vi "Talker.vi"(0 "Divide in":refnum<class "Divide.lvclass">, 5 "Subpanel Ref":refnum<vi>, 11 "Error In":errorcluster) -> (4 "Divide out":refnum<class "Divide.lvclass">, 15 "Error Out":errorcluster)   [LabVIEW 2020, in "Divide.lvclass"]
doc: "Method to call the UI Method. This will pass the object to the UI Method which will do the operation and return the object to the main vi."
uses:
  Divide.lvclass
  D:/Github Projects/LV_Assignment/Tasks/A18/A18/Classes/Arithmetic_Operations/Arithmetic_Operations.lvclass
  UI.vi
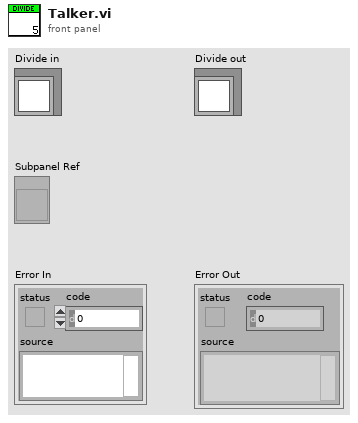
[diagram p1: front panel]
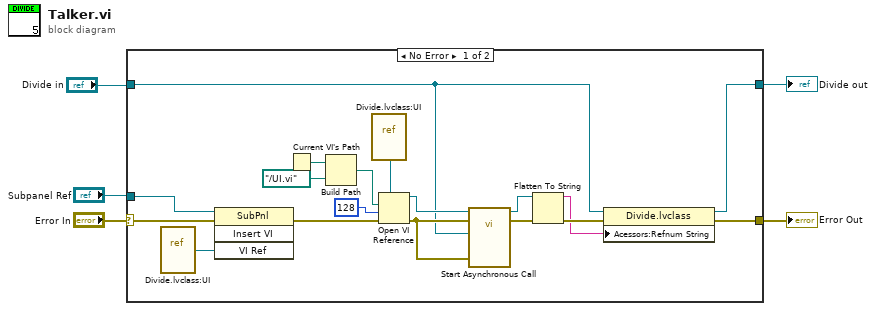
[diagram p0: block diagram]
diagram:
  n1 = case shown="No Error" "Error In" {
    selector: "Error In" -> [w21 w25]
    tunnel: [w13 w25] -> w4
    tunnel: [w12 w24] -> w2
    tunnel: "Divide in" -> [w11 w24]
    tunnel: "Subpanel Ref" -> [w19 _]
    frame No Error {
      n2 = vi-ref "Divide.lvclass:UI.vi"() -> (w10:refnum<vi>)
      n3 = invoke on="Invoke Node" class="SubPnl" method="Insert VI"(reference=w19, error in=w21, "VI Ref"=w10) -> (error out=w20:errorcluster)  [unwired: 1 in, 3 out]
      n4 = Current VI's Path() -> (path=w16:path)
      n5 = Build Path(base path=w16, name or relative path=path "../UI.vi") -> (appended path=w14:path)
      n6 = vi-ref "Divide.lvclass:UI.vi"() -> (w9:refnum<vi>)
      n7 = Open VI Reference(type specifier VI Refnum (for type only)=w9, vi path=w14, options=128, error in (no error)=w20) -> (vi reference=w18:refnum<vi>, error out=w23:errorcluster)  [unwired: 2 in]
      n8 = call-by-ref "Start Asynchronous Call"(reference=w18, error in=w23, "Divide in"=w11, "Error In"=w23) -> (reference out=w7:refnum<vi>, error out=w17:errorcluster)  [unwired: 11 in, 3 out]
      n9 = Flatten To String(anything=w7, error in (no error)=w17) -> (data string=w6:string, error out=w8:errorcluster)  [unwired: 2 in, 1 out]
      n10 = property class="Divide.lvclass"(reference=w11, error in=w8, "Acessors:Refnum String"=w6) -> (reference out=w12:refnum<class "Divide.lvclass">, error out=w13:errorcluster)
    }
    frame Error {
    }
  }
  "Divide out" <- w2
  "Error Out" <- w4
